vi "Msg Handler.vi"(6 "From Msg Event":bool, 9 "Msg":refnum<class "Msg.lvclass">, 10 "Actor in":refnum<class "Actor.lvclass">) -> (0 "Error out":errorcluster, 2 "Actor out":refnum<class "Actor.lvclass">)   [LabVIEW 2020, in "jettl.lvlib" / "Actor.lvlib"]
uses:
  Actor.lvlib
  Actor/Actor.lvclass
  Msg/Msg.lvclass
  Attributes/Attributes/Attributes.lvclass
  Error/Error.lvlib
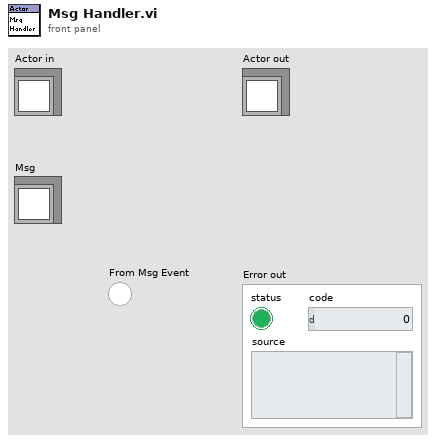
[diagram p1: front panel]
types:
  T1 = typedef "jettl.lvlib/Actor.lvlib/Msg Set.ctl" = set{refnum<class "Msg.lvclass">}
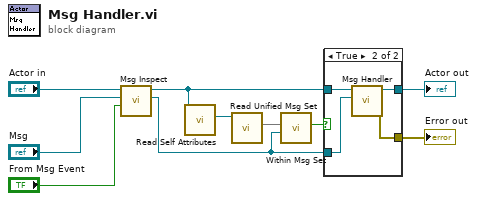
[diagram p0: block diagram]
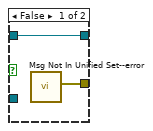
[diagram p2: hidden frame]
diagram:
  n1 = call-dynamic "Msg Inspect.vi"("From Msg Event"="From Msg Event", "Msg in"="Msg", "Actor in"="Actor in") -> ("Msg out"=w2:refnum<class "Msg.lvclass">, "Actor out"=w4:refnum<class "Actor.lvclass">)  [unwired: 7 in]
  n2 = call-dynamic "Read Self Attributes.vi"("Actor in"=w4) -> ("Self Attributes"=w10:refnum<class "Attributes.lvclass">)  [unwired: 10 in]
  n3 = call-dynamic "Read Unified Msg Set.vi"("Attributes in"=w10) -> ("Unified Msg Set"=w9:T1)  [unwired: 10 in]
  n4 = call "Within Msg Set.vi"("Msg"=w2, "Msg Set"=w9) -> ("Within Msg Set"=w8:bool)  [unwired: 9 in]
  n5 = case shown="True" w8 {
    tunnel: w4 -> [w12 w16]
    tunnel: [w12 w14] -> w7
    tunnel: w2 -> [_ w15]
    tunnel: [w11 w13] -> w6
    frame False {
      n6 = call "Msg Not In Unified Set--error.vi"() -> ("Error"=w11:errorcluster)  [unwired: 11 in]
    }
    frame True {
      n7 = call-dynamic "Msg Handler.vi"("Msg"=w15, "Actor in"=w16) -> ("Error out"=w13:errorcluster, "Actor out"=w14:refnum<class "Actor.lvclass">)  [unwired: 8 in]
    }
  }
  "Actor out" <- w7
  "Error out" <- w6
